vi "gigasealing_v7.vi"(0 "Pressure box control in":T3={"Pressure box COM"="", "pressure box type"=enum."Neuromatics", "High pos pressure (mBar)"=200.0, "Low pos pressure (mBar)"=80.0, "Vacuum pressure (mBar)"=-40.0, "calibration"=enum."Neuromatics"}, 1 "holding V (mV)":dbl=-70.0, 2 "Cm":dbl, 3 "Ra":dbl, 4 "apply suction":bool, 5 "gigasealing array":dbl[](array[numeric]), 6 "Slide Refnum":refnum<vi>, 7 "gigasealing options":T1={"atm wait (indices)"=10, "num samples for slope"=5, "delta suction (mbar)"=2.0, "if less than this slope, increase suction"=1.0, "else if less than this slope, maintain suction"=100.0, "else if less than this slope, decrease suction "=200.0, "max suction (mBar)"=-70.0}, 9 "Rm":dbl, 11 "GS timeout":i32=380, 12 "vhold applied?":bool, 13 "which manipulator":T2(ring)) -> (14 "set pressure":dbl, 15 "Vholding (mV)":dbl, 18 "vhold applied":bool, 19 "state out":T5=enum."Setting defaults...")   [LabVIEW 2015]
uses:
  controls/user_message_v6.ctl
  pipette cleaning/pressure box/cleaning_soft/controls/pressure_box_control.ctl
  pipette cleaning/pressure box/cleaning_soft/controls/pressure_box_type.ctl
panel:
  # "OUTPUTS"
  # "INPUTS"
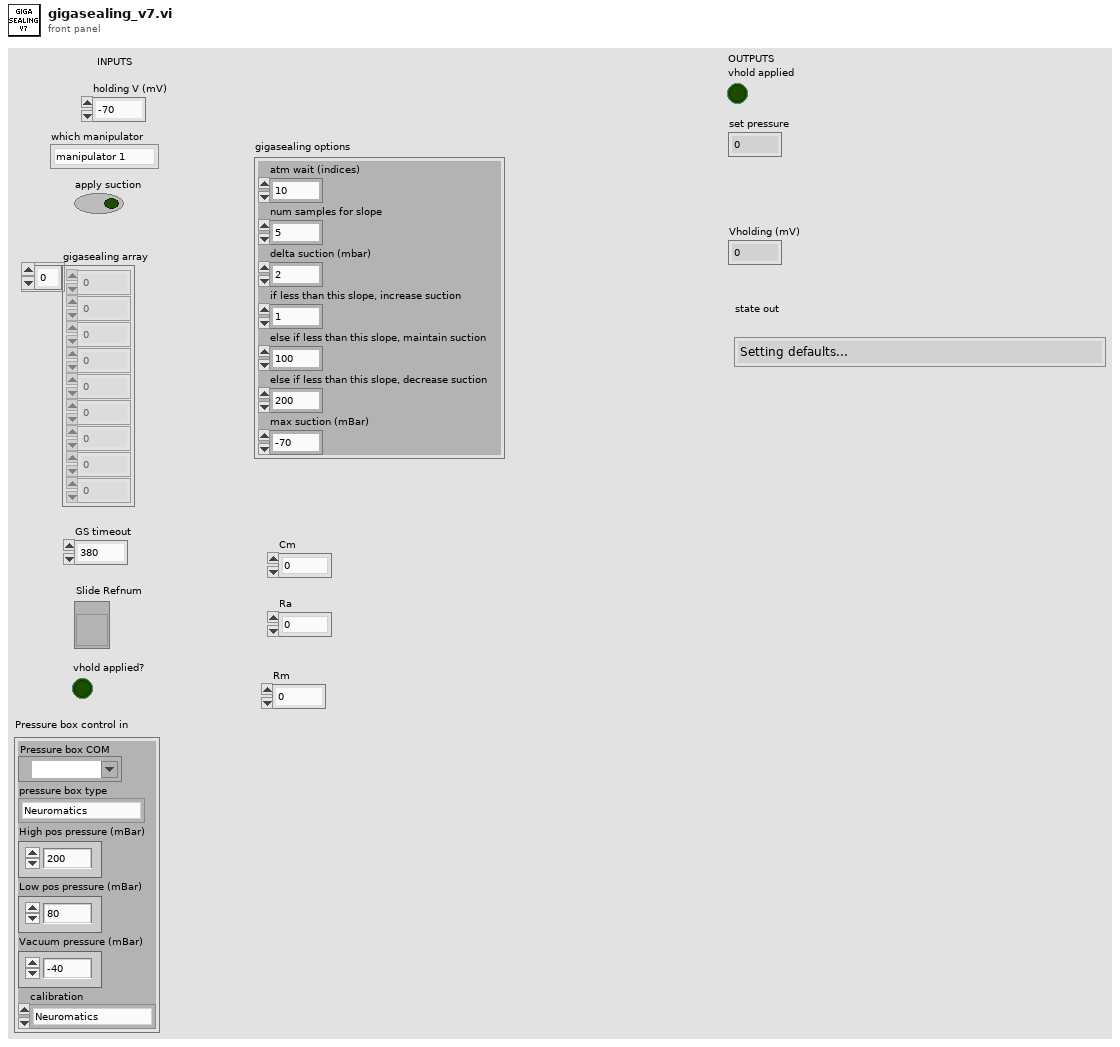
[diagram p1: front panel]
types:
  T1 = cluster{"atm wait (indices)":i32, "num samples for slope":i32, "delta suction (mbar)":dbl, "if less than this slope, increase suction":dbl, "else if less than this slope, maintain suction":dbl, "else if less than this slope, decrease suction ":dbl, "max suction (mBar)":dbl}
  T2 = enum16{"manipulator 1", "manipulator 2", "manipulator 3", "manipulator 4"}
  T3 = typedef "pressure_box_control.ctl" = cluster{"Pressure box COM":refnum<visa-resource-name>, "pressure box type":T4, "High pos pressure (mBar)":dbl, "Low pos pressure (mBar)":dbl, "Vacuum pressure (mBar)":dbl, "calibration":enum16{"PA_vacPump", "PA_venturi", "Neuromatics", "ilyaRig", "mightenRig"}}
  T4 = typedef "pressure_box_type.ctl" = enum16{"Neuromatics", "ProportionAir", "Demo box", "N-ProportionAir"}
  T5 = typedef "user_message_v6.ctl" = enum16{"Initializing...", "Setting defaults...", "Click OK to start patcherBot!", "Starting new attempt...", "Pipette repositioning...", "Initializing cell tracker...", "Gross approach...", "Human Positioning...", "In Process Calibration", "Detecting cell...", "Cell detected...", "Gigaseal Established...", "Breaking in...", "Successful breakin!", "Unsuccessful breakin!", "Whole-cell recording", "Saving autopatching parameters...", "Quitting VI", "Waiting for idle stage...", "Cleaning...", "Retracting pipette...", "DEBUG STATE", "Waiting to break in...", "Waiting for WC", "reclean", "Done with Current Set of Cells"}
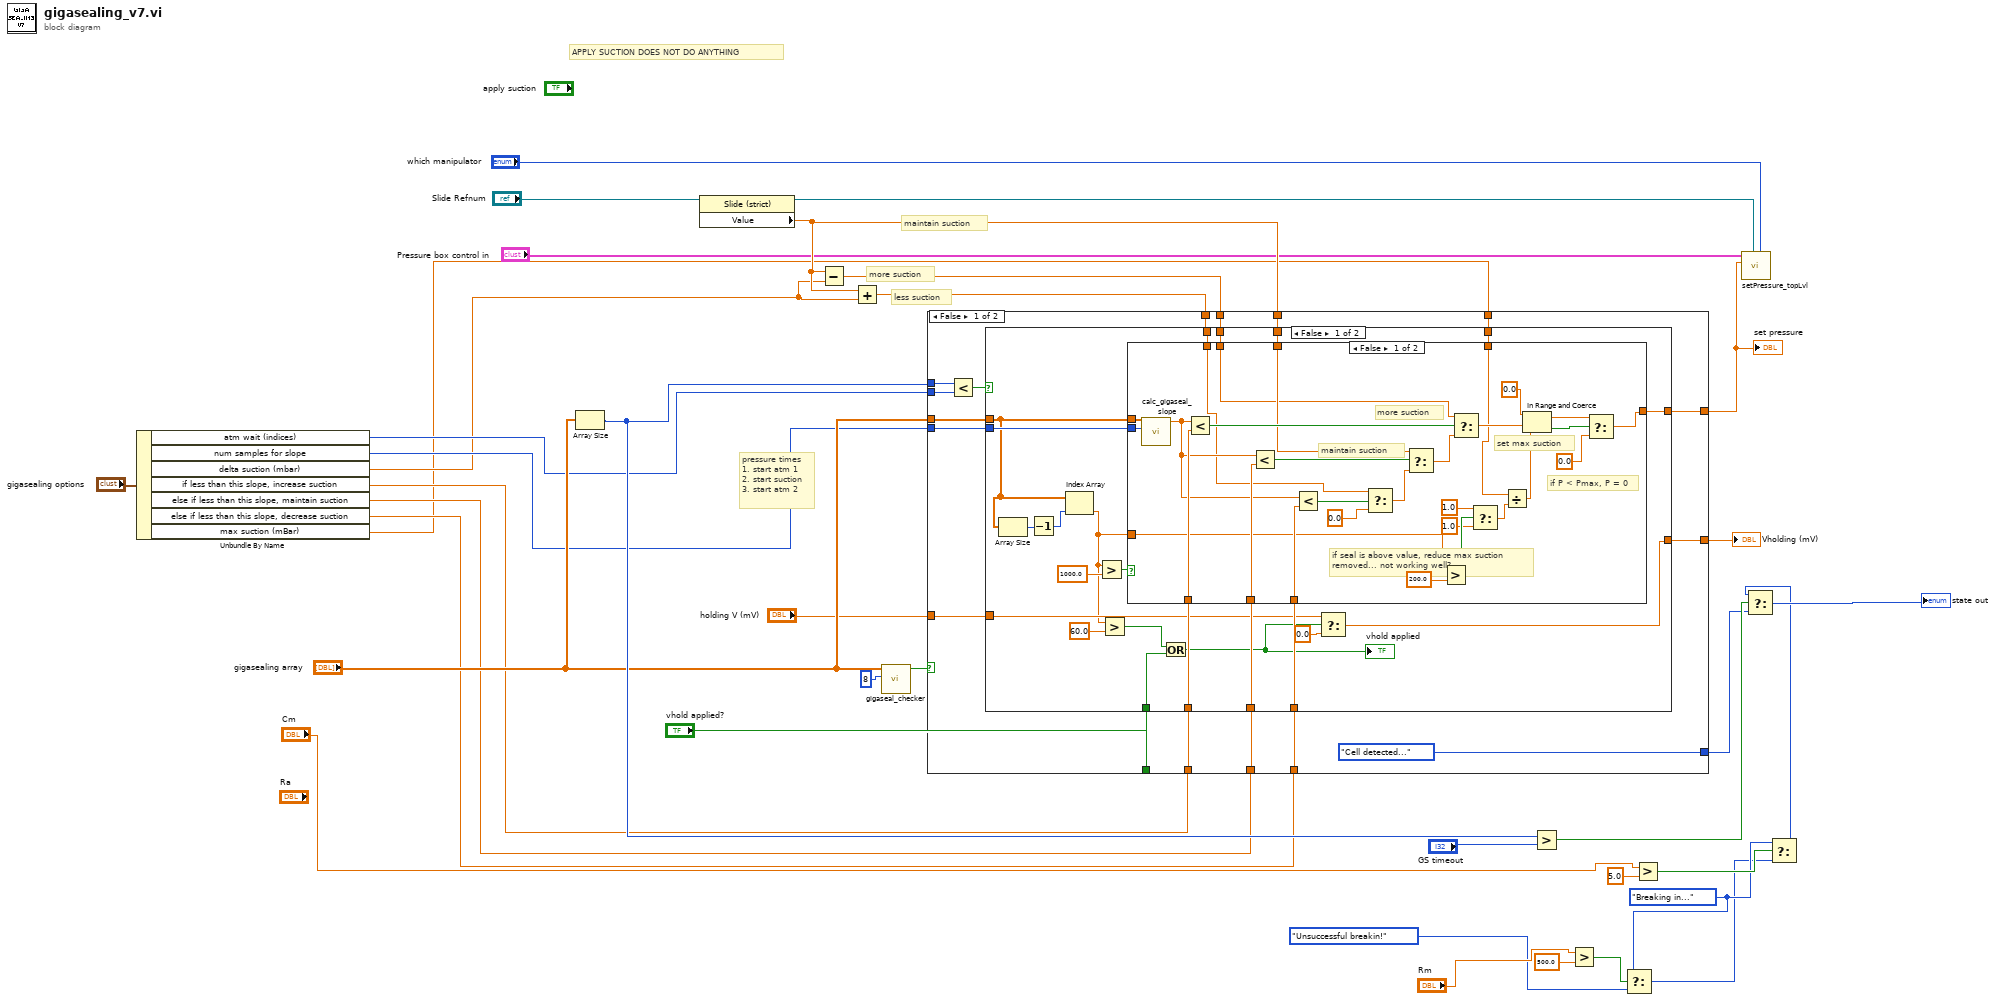
[diagram p0: block diagram]
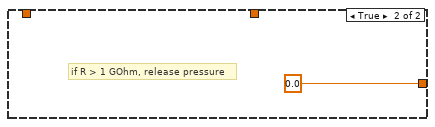
[diagram p2: hidden frame]
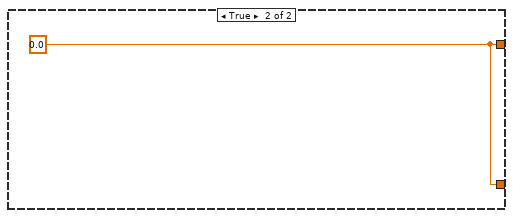
[diagram p3: hidden frame]
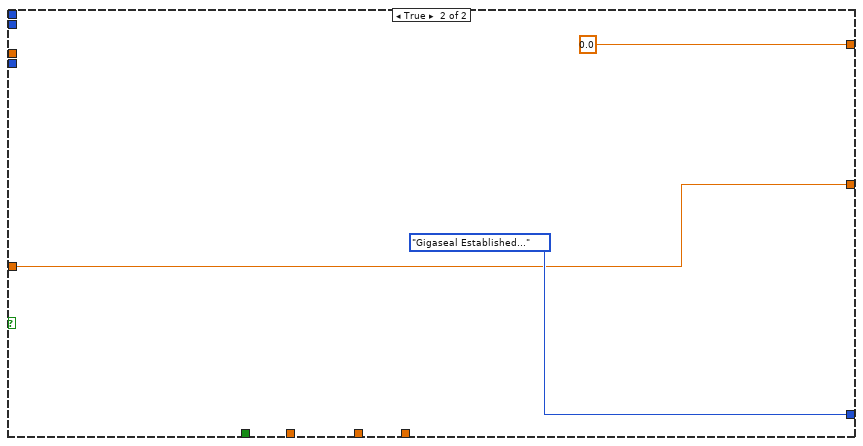
[diagram p4: hidden frame]
diagram:
  w3 = user_message_v6."Breaking in..." ("f")
  # "maintain suction"
  # "less suction"
  # "more suction"
  # "pressure times\n1. start atm 1\n2. start suction\n3. start atm 2"
  # "APPLY SUCTION DOES NOT DO ANYTHING"
  n1 = Unbundle By Name("gigasealing options") -> ("atm wait (indices)"=w17:i32, "num samples for slope"=w16:i32, "delta suction (mbar)"=w15:dbl, "if less than this slope, increase suction"=w14:dbl, "else if less than this slope, maintain suction"=w13:dbl, "else if less than this slope, decrease suction"=w12:dbl, "max suction (mBar)"=w11:dbl)
  n2 = Array Size(array="gigasealing array") -> (size(s)=w32:i32)
  n3 = property class="Slide (strict)"(reference="Slide Refnum") -> (reference out=w26:refnum<vi>, "Value"=w24:dbl)  [unwired: 1 in, 1 out]
  n4 = Subtract(x=w24, y=w15) -> (x-y=w25:dbl)
  n5 = Add(x=w24, y=w15) -> (x+y=w23:dbl)
  n6 = call "gigaseal_checker.vi"("num elements to look at"=8, "gigasealing array"="gigasealing array") -> ("Gigaseal?"=w28:bool)  [unwired: 9 in]
  n7 = case shown="False" w28 {
    tunnel: [w40 w108] -> w37
    tunnel: [user_message_v6."Cell detected..." ("state out") user_message_v6."Gigaseal Established..." ("state out")] -> w33
    tunnel: w32 -> [w53 _]
    tunnel: "gigasealing array" -> [w49 _]
    tunnel: w17 -> [w51 _]
    tunnel: [w50 0.0] -> w27
    tunnel: w16 -> [w48 _]
    tunnel: w14 -> [w47 _]
    tunnel: w25 -> [w46 _]
    tunnel: w13 -> [w45 _]
    tunnel: w24 -> [w44 _]
    tunnel: w12 -> [w43 _]
    tunnel: w23 -> [w42 _]
    tunnel: w11 -> [w41 _]
    tunnel: "holding V (mV)" -> [w39 w108]
    tunnel: "vhold applied?" -> [w38 _]
    frame False {
      n8 = Less?(x=w53, y=w51) -> (x < y?=w52:bool)
      n9 = case shown="False" w52 {
        tunnel: [w72 w107] -> w50
        tunnel: w49 -> [w66 _]
        tunnel: w48 -> [w76 _]
        tunnel: w47 -> [w75 _]
        tunnel: w46 -> [w74 _]
        tunnel: w45 -> [w73 _]
        tunnel: w44 -> [w71 _]
        tunnel: w43 -> [w70 _]
        tunnel: w42 -> [w69 _]
        tunnel: w41 -> [w63 _]
        tunnel: [w60 w107] -> w40
        tunnel: w39 -> [w59 _]
        tunnel: w38 -> [w56 _]
        frame False {
          n10 = Array Size(array=w66) -> (size(s)=w67:i32)
          n11 = Decrement(x=w67) -> (x-1=w68:i32)
          n12 = Index Array(array=w66, index=w68) -> (element=w55:dbl)
          n13 = Greater?(x=w55, y=1000.0) -> (0:w64:bool)
          n14 = Greater?(x=w55, y=60.0) -> (0:w58:bool)
          n15 = case shown="False" w64 {
            tunnel: w66 -> [w105 _]
            tunnel: w76 -> [w104 _]
            tunnel: w75 -> [w103 _]
            tunnel: w74 -> [w89 _]
            tunnel: w73 -> [w101 _]
            tunnel: [w85 0.0 ("f")] -> w72
            tunnel: w71 -> [w98 _]
            tunnel: w70 -> [w95 _]
            tunnel: w69 -> [w93 _]
            tunnel: w63 -> [w82 _]
            tunnel: w55 -> [w83 _]
            frame False {
              # "if seal is above value, reduce max suction\nremoved... not working well?"
              # "if P < Pmax, P = 0"
              # "set max suction"
              # "maintain suction"
              # "more suction"
              n16 = call "calc_gigaseal_slope.vi"("num samples"=w104, "gigasealing array"=w105) -> ("slope (Mohm / s)"=w94:dbl)  [unwired: 9 in]
              n17 = Less?(x=w94, y=w103) -> (x < y?=w102:bool)
              n18 = Less?(x=w94, y=w101) -> (x < y?=w99:bool)
              n19 = Less?(x=w94, y=w95) -> (x < y?=w96:bool)
              n20 = Select(t=w93, s=w96, f=0.0) -> (s? t:f=w97:dbl)
              n21 = Select(t=w98, s=w99, f=w97) -> (s? t:f=w100:dbl)
              n22 = Greater?(x=w83, y=200.0) -> (0:w79:bool)
              n23 = Select(t=w89, s=w102, f=w100) -> (s? t:f=w90:dbl)
              n24 = Select(t=1.0, s=w79, f=1.0) -> (s? t:f=w80:dbl)
              n25 = Divide(x=w82, y=w80) -> (x/y=w81:dbl)
              n26 = In Range and Coerce(upper limit=0.0, x=w90, lower limit=w81) -> (coerced(x)=w86:dbl, In Range?=w88:bool)
              n27 = Select(t=w86, s=w88, f=0.0) -> (s? t:f=w85:dbl)
            }
            frame True {
              # "if R > 1 GOhm, release pressure"
            }
          }
          n28 = Or(x=w58, y=w56) -> (x .or. y?=w57:bool)
          "vhold applied" <- w57
          n29 = Select(t=w59, s=w57, f=0.0) -> (s? t:f=w60:dbl)
        }
        frame True {
          w107 = 0.0
        }
      }
    }
    frame True {
    }
  }
  "Vholding (mV)" <- w37
  "set pressure" <- w27
  n30 = Greater?(x=w32, y="GS timeout") -> (0:w34:bool)
  n31 = Greater?(x="Rm", y=500.0) -> (0:w4:bool)
  n32 = Select(t=w3, s=w4, f=user_message_v6."Unsuccessful breakin!") -> (s? t:f=w1:T5)
  n33 = Greater?(x="Cm", y=5.0) -> (0:w7:bool)
  n34 = call "setPressure_topLvl.vi"("which manipulator"="which manipulator", "Slide Refnum"=w26, "set pressure (mBar)"=w27, "Pressure box control in"="Pressure box control in") -> ()  [unwired: 6 in, 2 out]
  n35 = Select(t=w3, s=w7, f=w1) -> (s? t:f=w10:T5)
  n36 = Select(t=w10, s=w34, f=w33) -> (s? t:f=→"state out":T5)
